vi "OS_Comm_to_Var_Analog.vi"(9 "Array":dbl[](array[numeric])) -> ()   [LabVIEW 2016, in "DNP3_Outstation_Template.lvlib"]
uses:
  DNP3_Outstation_Template.lvlib
  <vilib>/Utility/file.llb/Read Delimited Spreadsheet (string).vi
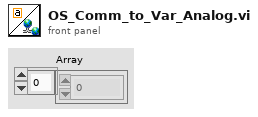
[diagram p1: front panel]
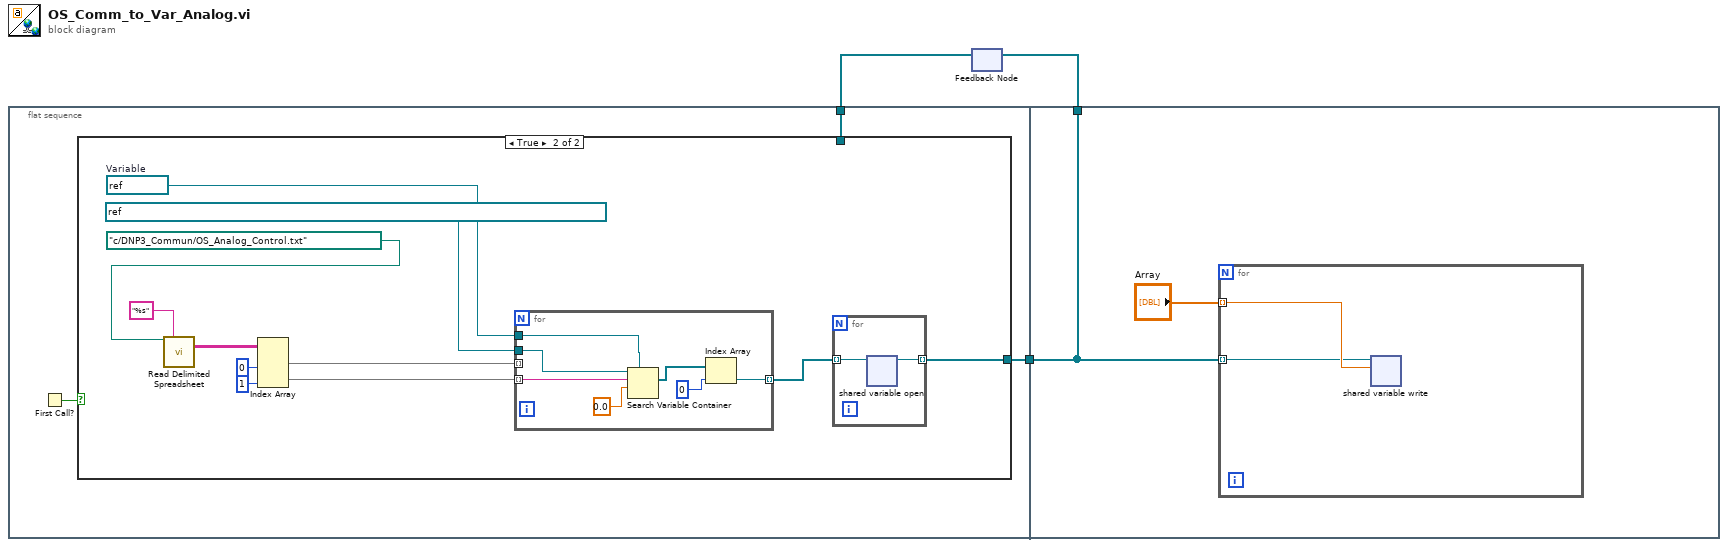
[diagram p0: block diagram]
diagram:
  n1 = flat-sequence {
    tunnel: [w5] -> w3
    tunnel: w1 -> [w4]
    tunnel: w3 -> [w28]
    tunnel: [w28] -> w2
    frame #0 {
      n2 = First Call?() -> (First Call?: T/F=w6:bool)
      n3 = case shown="True" w6 {
        tunnel: [w7 w8] -> w5
        tunnel: w4 -> [w7 _]
        frame False {
        }
        frame True {
          w10 = refnum<k21> refnum  # Variable
          n4 = call-poly <vilib>:"Read Delimited Spreadsheet.vi"("file path (dialog if empty)"=path "c:/DNP3_Commun/OS_Analog_Control.txt" ("file path (use dialog)"), "format (%s)"="%s") -> ("all rows"=w14:string[][])  [unwired: 8 in, 5 out]
          n5 = Index Array(array=w14, index (col) #1=0 ("disabled index (col)"), index (col) #2=1 ("index (col)")) -> (element #1=w17:string[], element #2=w18:string[])  [unwired: 2 in]
          n6 = for {
            tunnel: w10 -> [w25]
            tunnel: refnum<k21> "ni.var.psp://lc1 (bess)/DNP3_Outstation_Template/OS_Data_Variables/OS_Analog_Control" ("container refnum in") -> [w24]
            tunnel: w17 -> [_] mode=indexing
            tunnel: w18 -> [w23] mode=indexing
            tunnel: [w22] -> w9 mode=indexing
            n7 = Search Variable Container(7:w25, 9:0.0, 10:w23, 11:w24) -> (2:w27:refnum<k21>[])  [unwired: 2 in, 2 out]
            n8 = Index Array(array=w27, index=0) -> (element=w22:refnum<k21>)
          }
          n9 = for {
            tunnel: w9 -> [w20] mode=indexing
            tunnel: [w19] -> w8 mode=indexing
            n10 = shared-variable-open(w20) -> (w19:refnum<k21>)  [unwired: 2 in, 1 out]
          }
        }
      }
    }
    frame #1 {
      n11 = for {
        tunnel: "Array" -> [w31] mode=indexing
        tunnel: w28 -> [w30] mode=indexing
        n12 = shared-variable-write(w30, w31) -> ()  [unwired: 1 in, 2 out]
      }
    }
  }
  n13 = feedback-in #1(w2) -> ()
  n14 = feedback #1() -> (w1:refnum<k21>[])  [unwired: 1 in]
